vi "Out_S1F12.vi"(8 "error in (no error)":errorcluster, 10 "S1F12":T1, 11 "S1 Message Class in":refnum<class "S1 Message Class.lvclass">) -> (0 "error out":errorcluster, 3 "S1 Message Class out":refnum<class "S1 Message Class.lvclass">)   [LabVIEW 2020, in "SECS Communication.lvlib" / "S1 Message Class.lvclass"]
uses:
  S1 Message Class.lvclass
  D:/Dropbox/SECS/LabVIEW Code/Com/SECS Communication/SECS-II Class/SECS-II Class.lvclass
  S1F12.ctl
  SECS-II Class/Data Message_List.vi
  SECS-II Class/Data Message_U4.vi
  SECS-II Class/Data Message_ASCII.vi
  S1 Message Class.lvclass/S1 Message Class.ctl
  SECS-II Class/SECS-II Class.lvclass
  D:/Dropbox/SECS/LabVIEW Code/Com/SECS Communication/S1 Message Class/S1 Message Class.lvclass
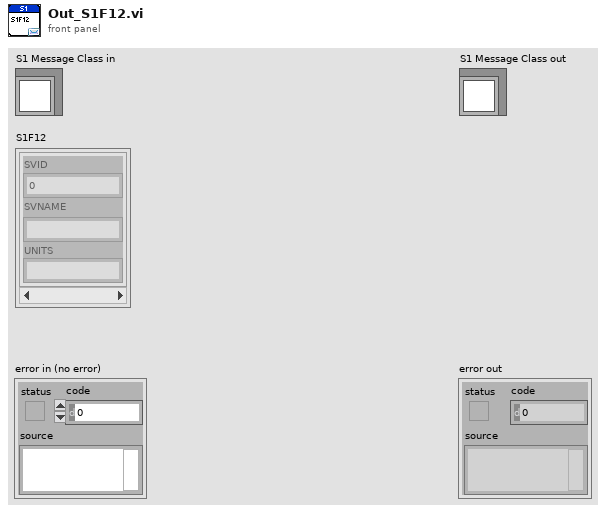
[diagram p1: front panel]
types:
  T1 = typedef "SECS Communication.lvlib/S1 Message Class.lvclass/S1F12.ctl" = cluster{"SVID":u32, "SVNAME":string, "UNITS":string}[]
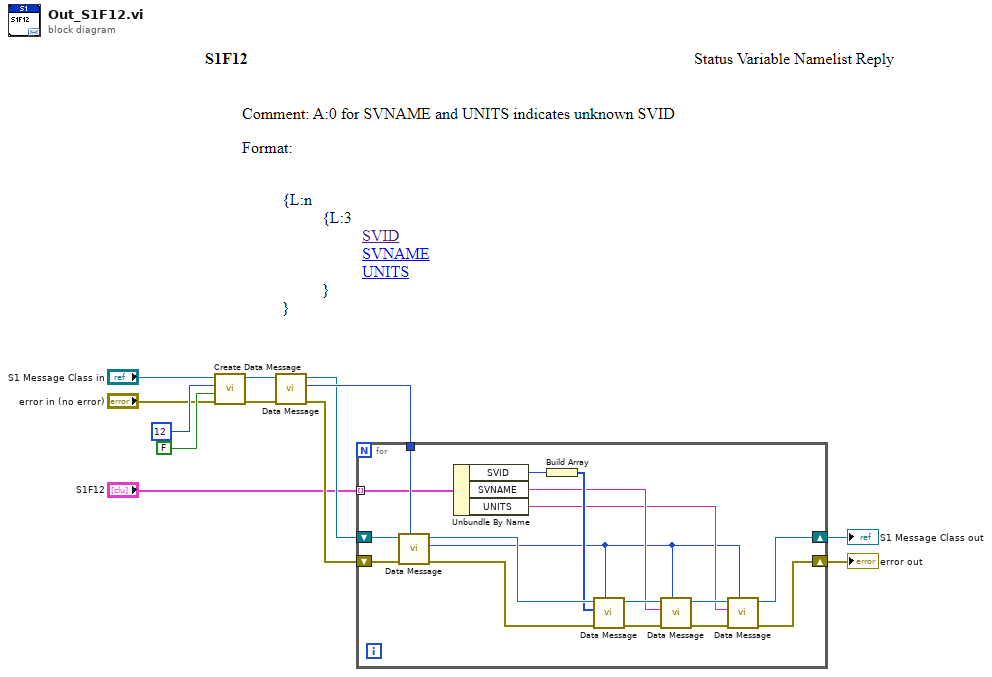
[diagram p0: block diagram]
diagram:
  n1 = call "Create Data Message.vi"("error in (no error)"="error in (no error)", "W-Bit"=FALSE, "Function"=u8 12, "SECS-II Class in"="S1 Message Class in") -> ("error out"=w8:errorcluster, "SECS-II Class out"=w9:refnum<class "S1 Message Class.lvclass">)  [unwired: 6 in]
  n2 = call-poly "Data Message.vi"("error in"=w8, "SECS-II Class in"=w9) -> ("error out"=w7:errorcluster, "Index"=w10:i32, "SECS-II Class out"=w6:refnum<class "S1 Message Class.lvclass">)  [unwired: 7 in]
  n3 = for {
    tunnel: w10 -> [w27]
    shift-right: [w13] -> w3
    shift-left: w7 -> [w28]
    shift-right: [w14] -> w2
    shift-left: w6 -> [w29]
    tunnel: "S1F12" -> [w24] mode=indexing
    n4 = call-poly "Data Message.vi"("Parent Index"=w27, "error in"=w28, "SECS-II Class in"=w29) -> ("error out"=w26:errorcluster, "Index"=w15:i32, "SECS-II Class out"=w25:refnum<class "S1 Message Class.lvclass">)  [unwired: 6 in]
    n5 = Unbundle By Name(w24) -> ("SVID"=w23:u32, "SVNAME"=w19:string, "UNITS"=w16:string)
    n6 = Build Array(w23) -> (w22:u32[])
    n7 = call-poly "Data Message.vi"("Parent Index"=w15, "error in"=w26, "Data"=w22, "SECS-II Class in"=w25) -> ("error out"=w20:errorcluster, "SECS-II Class out"=w21:refnum<class "S1 Message Class.lvclass">)  [unwired: 6 in]
    n8 = call-poly "Data Message.vi"("Parent Index"=w15, "error in"=w20, "Data"=w19, "SECS-II Class in"=w21) -> ("error out"=w17:errorcluster, "SECS-II Class out"=w18:refnum<class "S1 Message Class.lvclass">)  [unwired: 6 in]
    n9 = call-poly "Data Message.vi"("Parent Index"=w15, "error in"=w17, "Data"=w16, "SECS-II Class in"=w18) -> ("error out"=w13:errorcluster, "SECS-II Class out"=w14:refnum<class "S1 Message Class.lvclass">)  [unwired: 6 in]
  }
  "error out" <- w3
  "S1 Message Class out" <- w2
